vi "Do_channel_mathsPLL.vi"(4 "Output Index":i32, 5 "Channel Values In":string[][](array[string]), 6 "Channel Names":string[](array[string]), 7 "Maths Equation":string) -> (0 "Error String":string, 1 "Channel Values Out":string[][](array[string]), 3 "Results":dbl[](array[numeric]) format="%0.2f")   [LabVIEW 2021]
uses:
  <vilib>/Utility/error.llb/whitespace.ctl
  Globals/ParallelExecutionGlobal.vi
  Data_plotting_vis/Results_plotter_Global.vi
  <vilib>/gmath/NI_Gmath.lvlib
panel:
  out "Numeric":i32
  out "Array":string[](array[string])
  out "Generic Equation":string
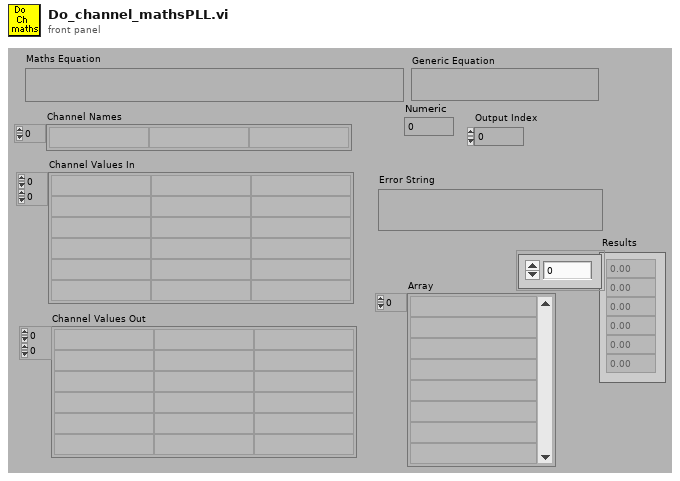
[diagram p1: front panel]
types:
  T1 = cluster{"Tables":i32[][], "Y Values":dbl[], "Variables input decode":i32[], i32[]}[]
  T2 = cluster{"Y Values":dbl[][], "Tables":i32[][][], "Variables input decode":i32[], "Variables output decode":i32[]}
  T3 = cluster{"Tables":i32[][], "Y Values":dbl[], "Variables input decode":i32[], i32[]}
  T4 = typedef "whitespace.ctl" = u16
  T5 = typedef "LVDateTimeRec.ctl" = cluster{"fractional second":dbl, "second":i32, "minute":i32, "hour":i32, "day of month":i32, "month":i32, "year":i32, "day of week":i32, "day of year":i32, "DST":i32}
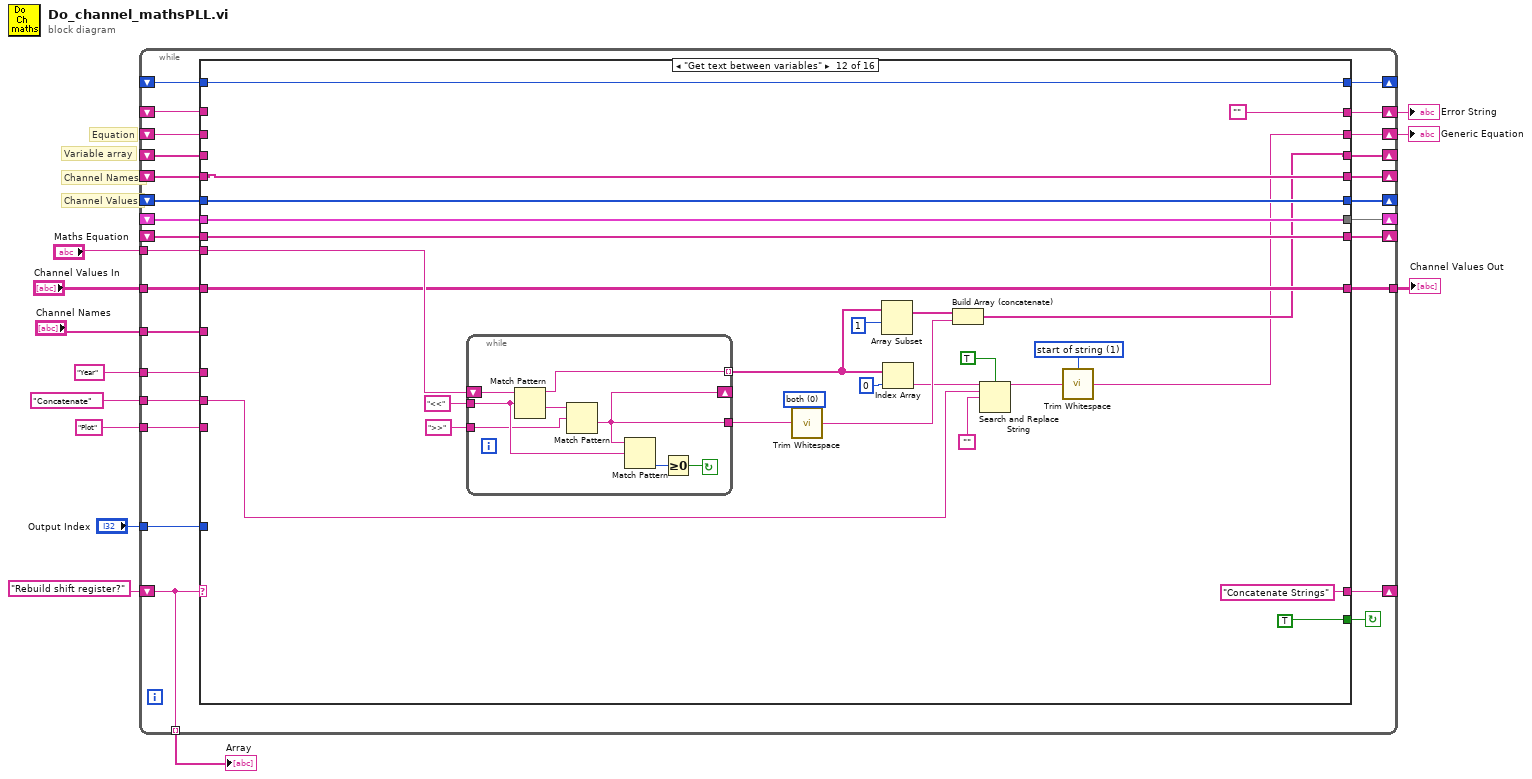
[diagram p0: block diagram]
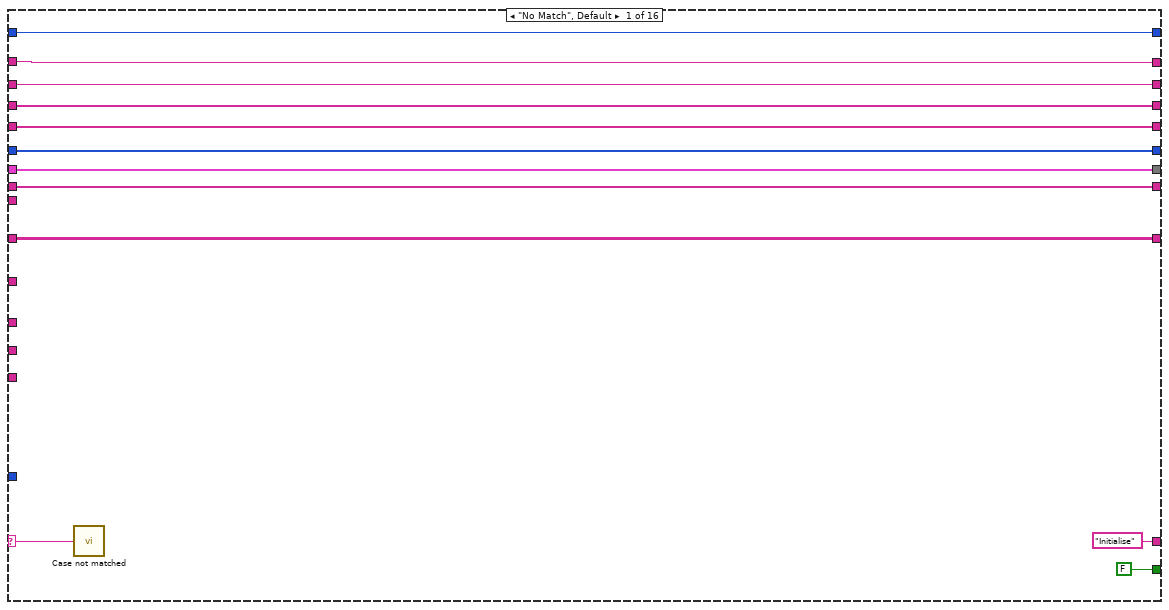
[diagram p2: hidden frame]
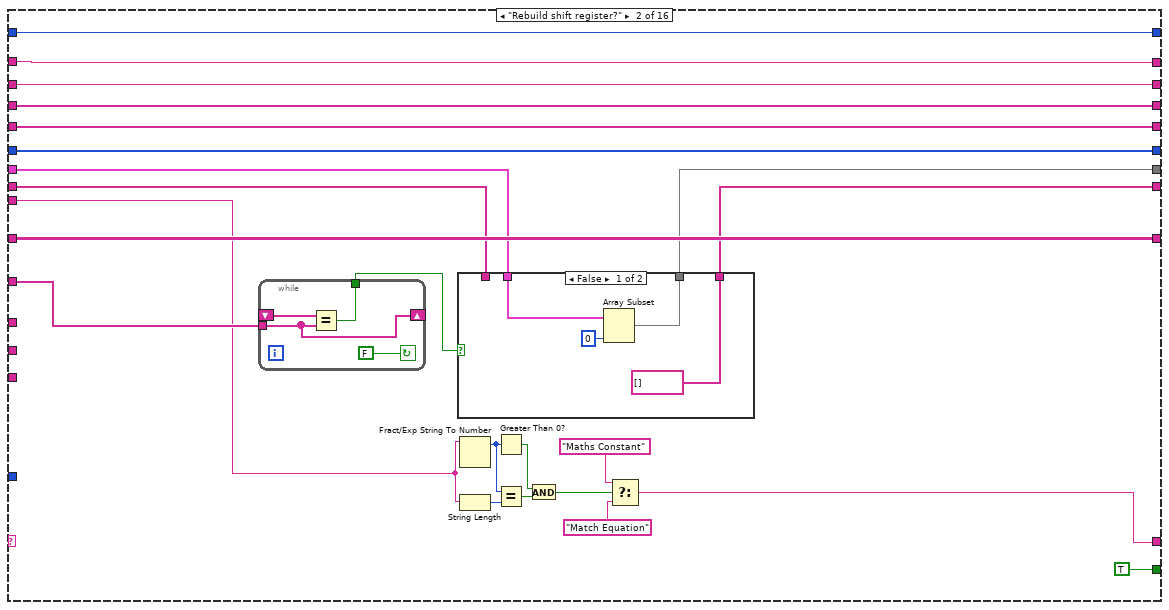
[diagram p3: hidden frame]
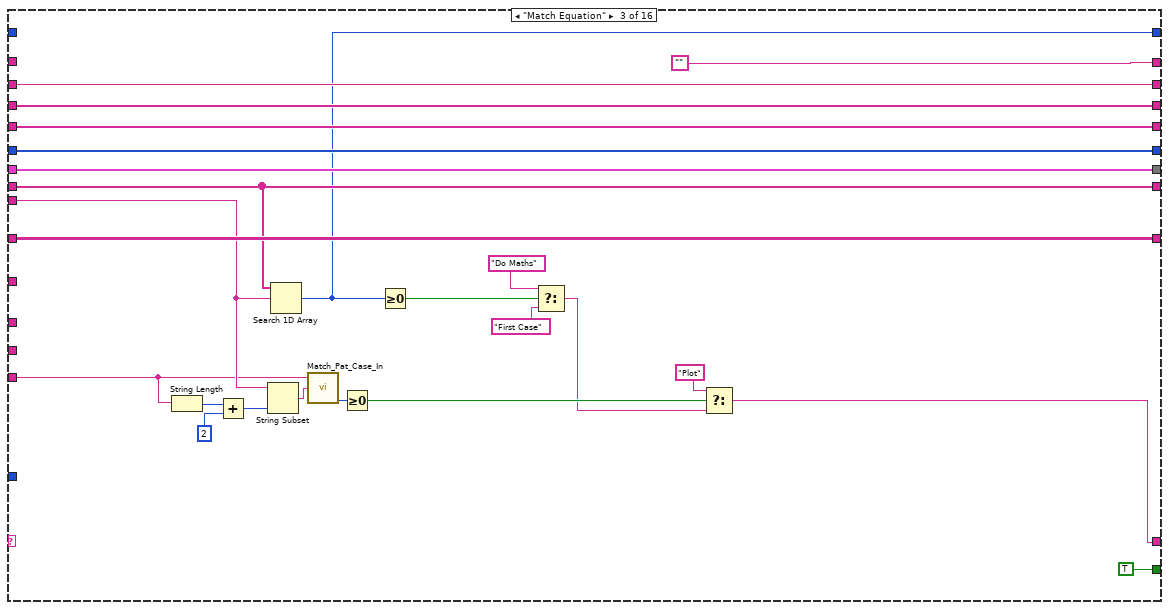
[diagram p5: hidden frame]
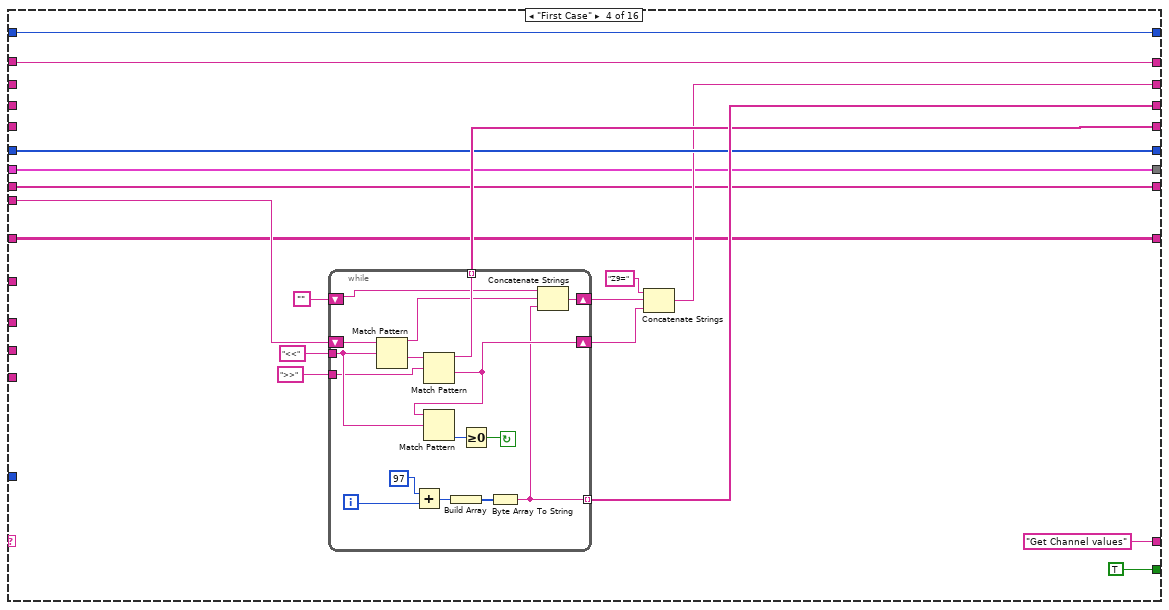
[diagram p6: hidden frame]
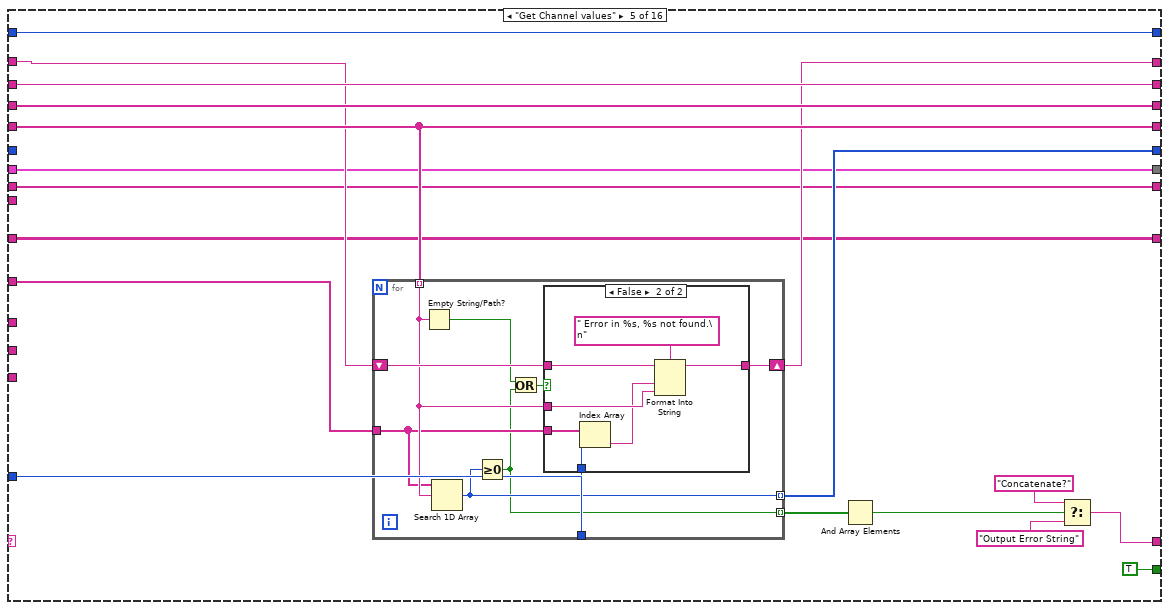
[diagram p7: hidden frame]
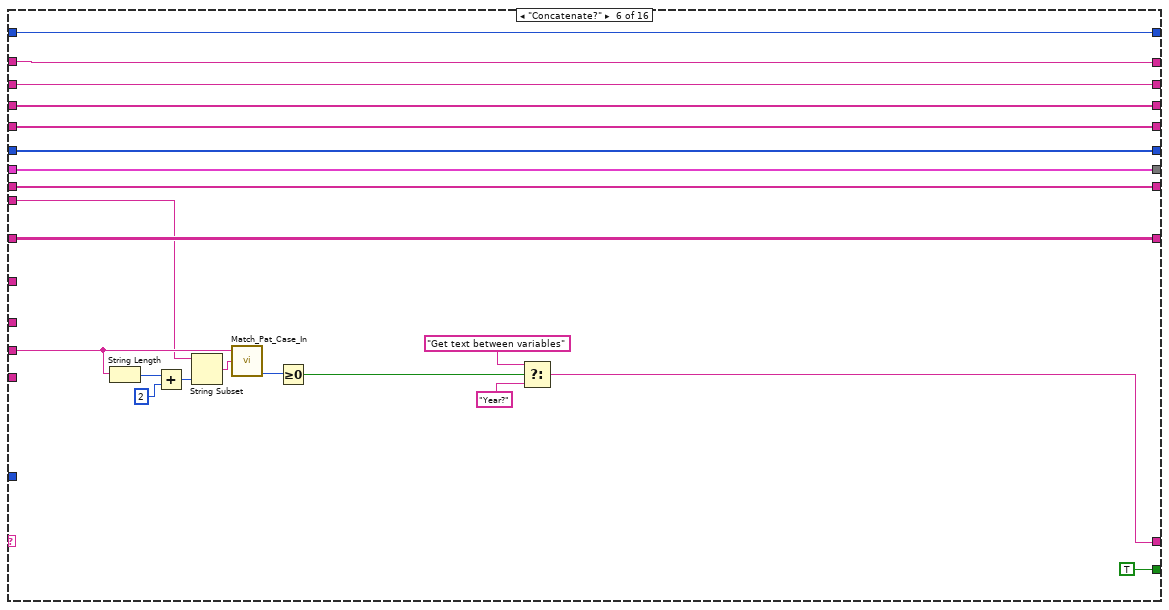
[diagram p9: hidden frame]
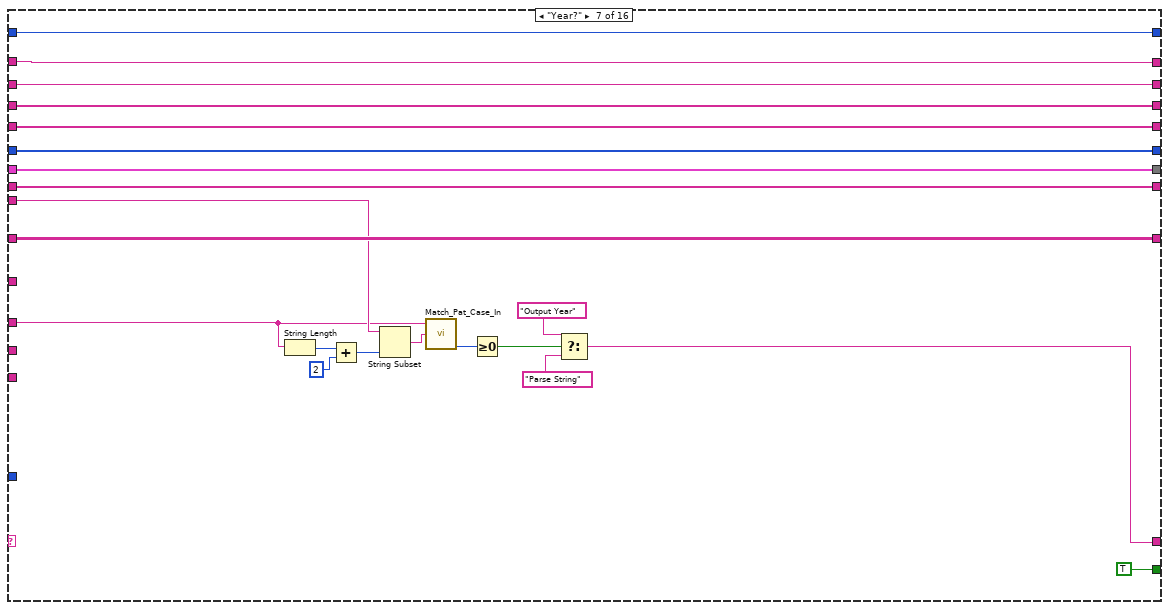
[diagram p10: hidden frame]
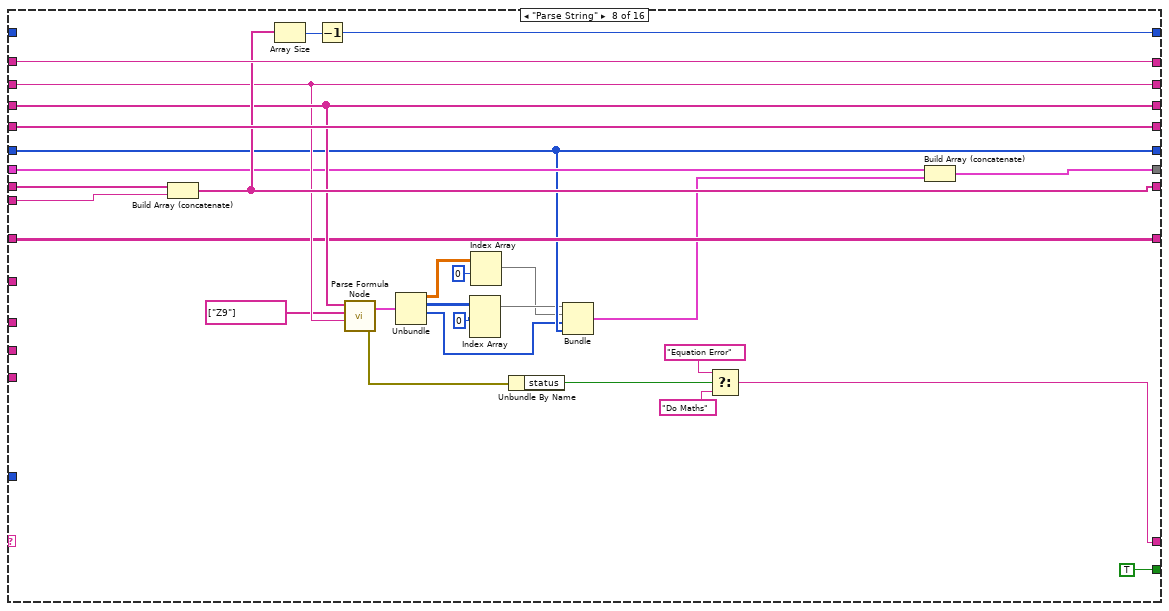
[diagram p11: hidden frame]
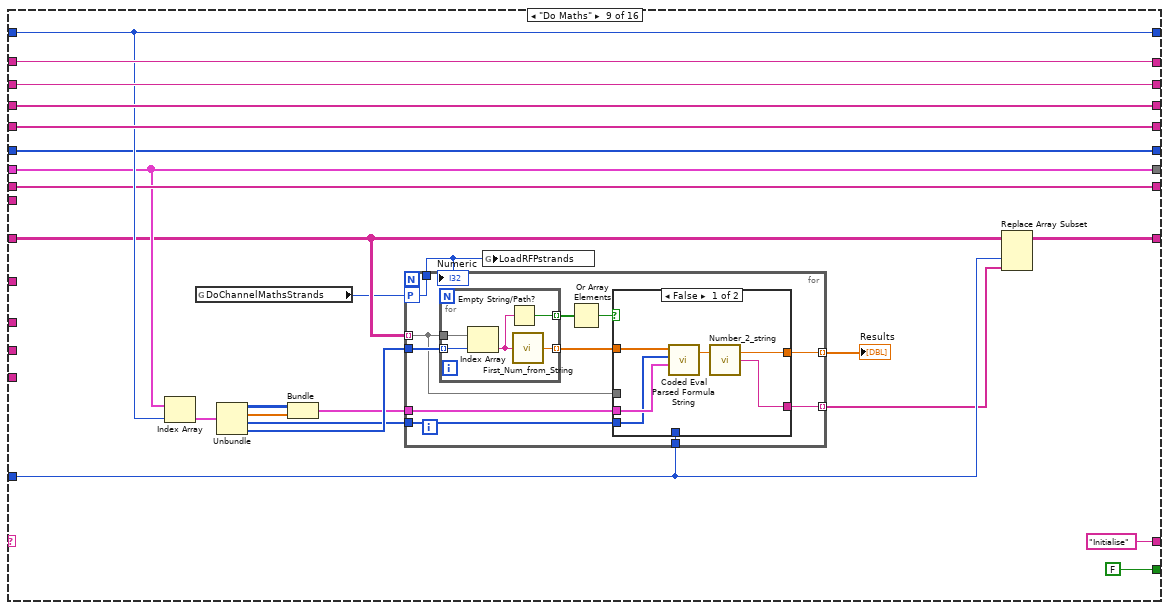
[diagram p12: hidden frame]
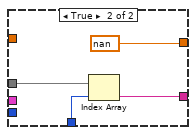
[diagram p13: hidden frame]
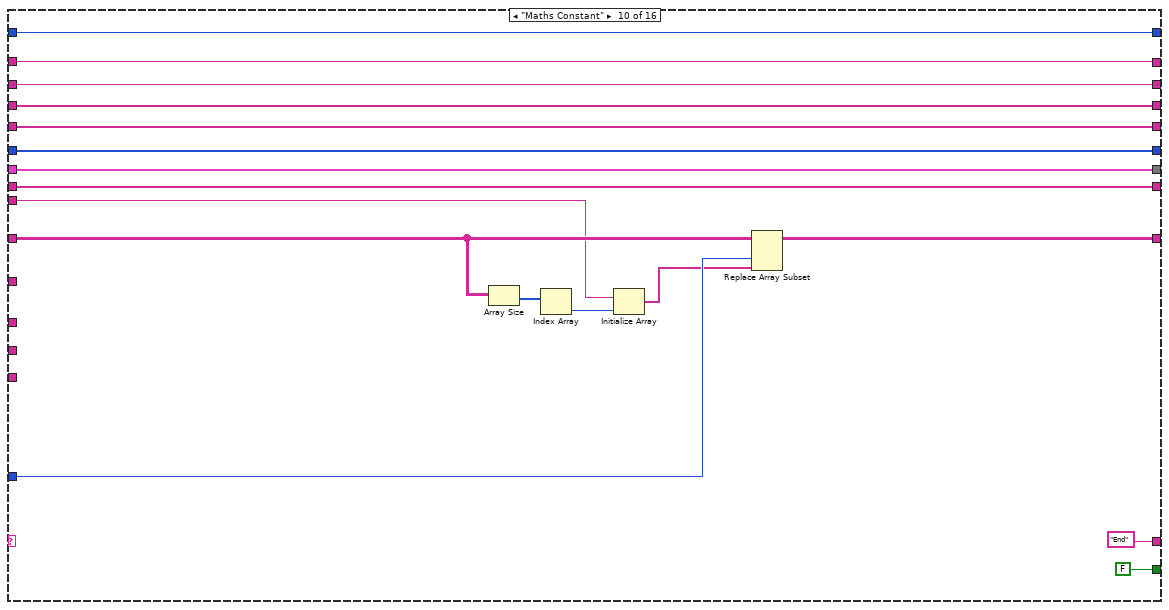
[diagram p14: hidden frame]
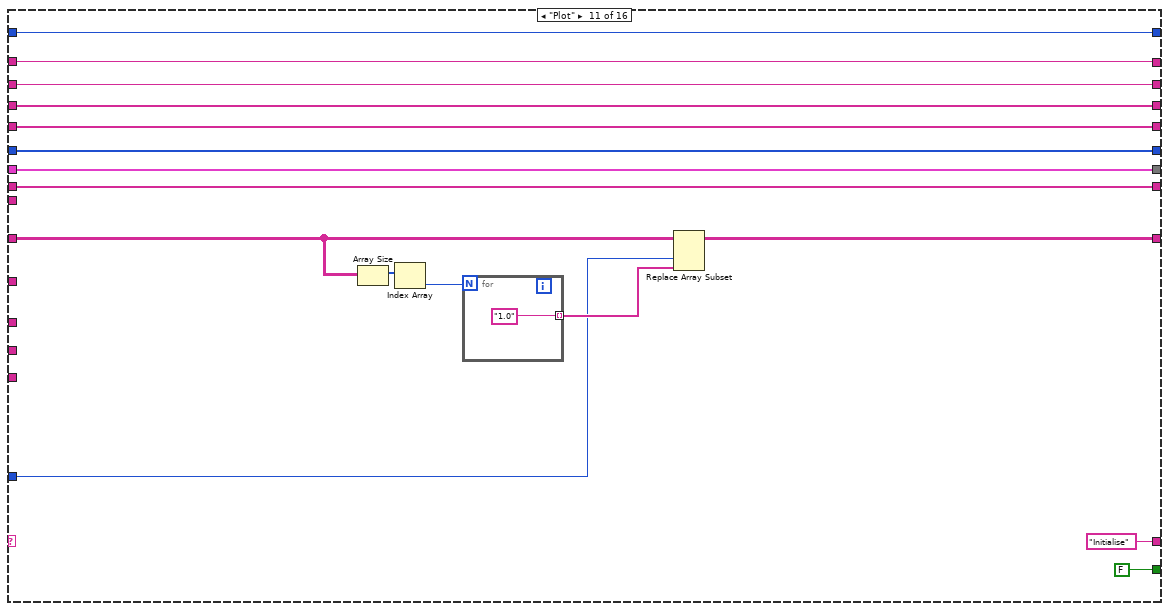
[diagram p15: hidden frame]
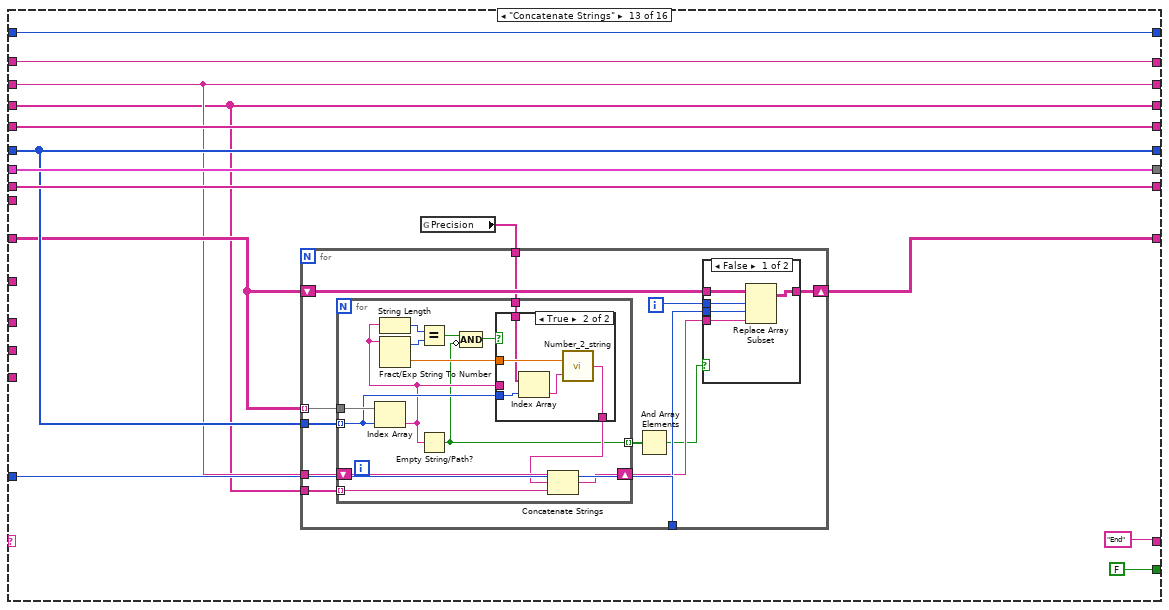
[diagram p16: hidden frame]
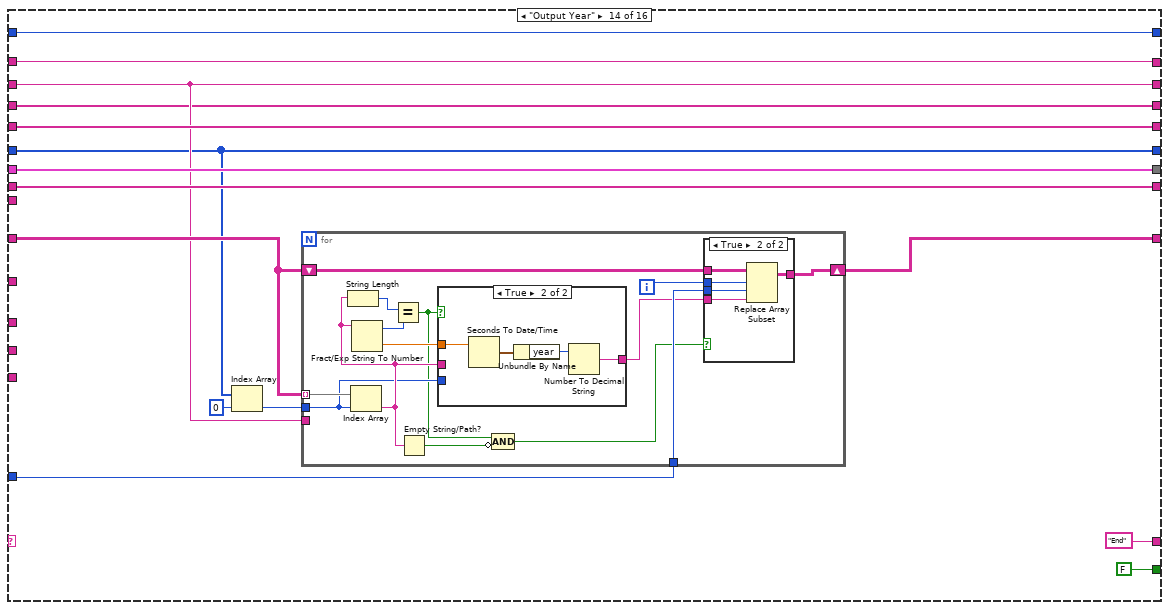
[diagram p19: hidden frame]
diagram:
  # "Channel Names"
  # "Variable array"
  # "Channel Values"
  # "Equation"
  n1 = while {
    tunnel: [w17] -> w6
    tunnel: "Output Index" -> [w18]
    shift-left: _ -> [w19]
    shift-right: [w20] -> _
    shift-left: _ -> [w23]
    shift-right: [w22] -> _
    shift-left: _ -> [w21]
    shift-right: [w24] -> _
    tunnel: "Channel Values In" -> [w25]
    tunnel: "Channel Names" -> [w26]
    tunnel: "Maths Equation" -> [w27]
    shift-left: _ -> [w29]
    shift-right: [w28] -> _
    shift-left: _ -> [w31]
    shift-right: [w30] -> _
    shift-left: _ -> [w33]
    shift-right: [w32] -> _
    shift-left: _ -> [w35]
    shift-right: [w34] -> w8
    shift-left: _ -> [w37]
    shift-right: [w36] -> w9
    shift-left: "Rebuild shift register?" -> [w13]
    shift-right: [w38] -> _
    tunnel: "Concatenate" ("regular expression") -> [w16]
    tunnel: "Plot" ("regular expression") -> [w15]
    tunnel: "Year" ("regular expression") -> [w14]
    tunnel: [w13] -> w1 mode=indexing
    stop <- w39 continue-if-true
    n2 = case shown="\"Get text between variables\"" w13 {
      selector: w13 -> [w40 _ _ _ _ _ _ _ _ _ _ _ _ _ _ _]
      tunnel: [FALSE TRUE TRUE TRUE TRUE TRUE TRUE TRUE FALSE FALSE FALSE TRUE FALSE FALSE TRUE FALSE] -> w39
      tunnel: ["Initialise" w53 w86 "Get Channel values" w145 w178 w208 w234 "Initialise" "End" "Initialise" "Concatenate Strings" "End" "End" "Output Error String" "Initialise"] -> w38
      tunnel: w37 -> [w49 w73 _ w111 w153 w198 w219 w246 w268 w310 w326 _ w376 w429 w459 w472]
      tunnel: [w49 w73 "" w111 w154 w198 w219 w246 w268 w310 w326 "" w376 w429 w458 w472] -> w36
      tunnel: w35 -> [w48 w72 w108 _ w159 w197 w218 w242 w266 w308 w324 _ w368 w422 w461 w482]
      tunnel: [w48 w72 w108 w116 w159 w197 w218 w242 w266 w308 w324 w332 w368 w422 w461 w482] -> w34
      tunnel: w33 -> [w47 w71 w107 _ w158 w196 w217 w243 w267 w309 w325 _ w367 w421 w468 w483]
      tunnel: [w47 w71 w107 w123 w158 w196 w217 w243 w267 w309 w325 w343 w367 w421 w468 w483] -> w32
      tunnel: w31 -> [w46 w70 w106 _ w156 w195 w216 w247 w269 w311 w327 w348 w377 w430 w469 w484]
      tunnel: [w46 w70 w106 w119 w156 w195 w216 w247 w269 w311 w327 w348 w377 w430 w469 w484] -> w30
      tunnel: w29 -> [w45 w69 w105 w118 _ w194 w215 w233 w259 w304 w320 w353 w372 w420 w464 w476]
      tunnel: [w45 w69 w105 w118 w155 w194 w215 w233 w259 w304 w320 w353 w372 w420 w464 w476] -> w28
      tunnel: w27 -> [_ w52 w92 w124 _ w182 w202 w220 _ w298 _ w355 _ _ w460 _]
      tunnel: w26 -> [_ w66 _ _ w157 _ _ _ _ _ _ _ _ _ _ w474]
      tunnel: w25 -> [w41 w67 w103 w112 w149 w189 w207 w238 w251 w301 w316 w349 w371 w425 w463 w475]
      tunnel: [w44 w64 w104 w115 w152 w193 w214 w239 w263 w305 w321 w352 w373 w426 w465 w479] -> w24
      tunnel: w23 -> [w43 w62 w102 w114 w151 w192 w213 w245 w264 w306 w322 w351 w374 w427 w466 w480]
      tunnel: [w43 w61 w102 w114 w151 w192 w213 w244 w264 w306 w322 w351 w374 w427 w466 w480] -> w22
      tunnel: w21 -> [w44 w63 w104 w115 w152 w193 w214 w241 w263 w305 w321 w352 w373 w426 w465 w479]
      tunnel: [w42 w68 w101 w113 w150 w191 w212 w240 w265 w307 w323 w350 w375 w428 w467 w481] -> w20
      tunnel: w19 -> [w42 w68 _ w113 w150 w191 w212 _ w265 w307 w323 w350 w375 w428 w467 w481]
      tunnel: w18 -> [_ _ _ _ w143 _ _ _ w257 w302 w317 _ w370 w424 _ w478]
      tunnel: [w41 w67 w103 w112 w149 w189 w207 w238 w258 w303 w319 w349 w369 w423 w463 w477] -> w17
      tunnel: w16 -> [_ _ _ _ _ w188 _ _ _ _ _ w337 _ _ _ _]
      tunnel: w15 -> [_ _ w91 _ _ _ _ _ _ _ _ _ _ _ _ _]
      tunnel: w14 -> [_ _ _ _ _ _ w199 _ _ _ _ _ _ _ _ _]
      frame "No Match", Default {
        n3 = call "Case not matched.vi"("Case Name not Matched"=w40) -> ()
      }
      frame "Rebuild shift register?" {
        n4 = while {
          shift-right: [w83] -> _
          shift-left: _ -> [w84]
          tunnel: w66 -> [w83]
          tunnel: [w82] -> w65
          stop <- FALSE continue-if-true
          n5 = Equal?(x=w84, y=w83) -> (x = y?=w82:bool)
        }
        n6 = case shown="False" w65 {
          tunnel: [w76 w80] -> w64
          tunnel: w63 -> [w78 w80]
          tunnel: w62 -> [_ w79]
          tunnel: [string[] [] w79] -> w61
          frame False {
            n7 = Array Subset(array=w78, length=0) -> (w76:T1)  [unwired: 1 in]
          }
          frame True {
          }
        }
        n8 = Fract/Exp String To Number(string=w52) -> (offset past number=w60:i32)  [unwired: 3 in, 1 out]
        n9 = String Length(string=w52) -> (length=w59:i32)
        n10 = Greater Than 0?(x=w60) -> (x > 0?=w57:bool)
        n11 = Equal?(x=w60, y=w59) -> (x = y?=w58:bool)
        n12 = And(x=w57, y=w58) -> (x .and. y?=w56:bool)
        n13 = Select(t="Maths Constant", s=w56, f="Match Equation") -> (s? t:f=w53:string)
      }
      frame "Match Equation" {
        n14 = String Length(string=w91) -> (length=w93:i32)
        n15 = Add(x=w93, y=2) -> (x+y=w95:i32)
        n16 = String Subset(string=w92, length (rest)=w95) -> (substring=w96:string)  [unwired: 1 in]
        n17 = Search 1D Array(1D array=w102, element=w92) -> (index of element=w101:i32)  [unwired: 1 out]
        n18 = call "Match_Pat_Case_In.vi"("String to match"=w91, "String"=w96) -> ("offset past match"=w89:i32)  [unwired: 1 in, 3 out]
        n19 = Greater Or Equal To 0?(x=w89) -> (x >= 0?=w88:bool)
        n20 = Greater Or Equal To 0?(x=w101) -> (x >= 0?=w100:bool)
        n21 = Select(t="Do Maths", s=w100, f="First Case") -> (s? t:f=w87:string)
        n22 = Select(t="Plot", s=w88, f=w87) -> (s? t:f=w86:string)
      }
      frame "First Case" {
        n23 = while {
          shift-left: "" -> [w129]
          shift-right: [w130] -> w121
          tunnel: [w131] -> w123 mode=indexing
          tunnel: [w137] -> w119 mode=indexing
          shift-left: w124 -> [w142]
          shift-right: [w140] -> w120
          tunnel: "<<" ("regular expression") -> [w128]
          tunnel: ">>" ("regular expression") -> [w127]
          i -> [w133]
          stop <- w138 continue-if-true
          n24 = Match Pattern(string=w142, regular expression=w128) -> (before substring=w132:string, after substring=w141:string)  [unwired: 3 out]
          n25 = Add(x=97, y=w133) -> (x+y=w135:i32)
          n26 = Match Pattern(string=w141, regular expression=w127) -> (before substring=w137:string, after substring=w140:string)  [unwired: 3 out]
          n27 = Match Pattern(string=w140, regular expression=w128) -> (offset past match=w139:i32)  [unwired: 4 out]
          n28 = Build Array(w135) -> (w136:i32[])
          n29 = Greater Or Equal To 0?(x=w139) -> (x >= 0?=w138:bool)
          n30 = Byte Array To String(unsigned byte array=w136) -> (string=w131:string)
          n31 = Concatenate Strings(w129, w132, w131) -> (w130:string)
        }
        n32 = Concatenate Strings("Z9=" ("Substring"), w121, w120) -> (w116:string)
      }
      frame "Get Channel values" {
        n33 = for {
          tunnel: w157 -> [w164]
          tunnel: w156 -> [w166] mode=indexing
          tunnel: [w167] -> w155 mode=indexing
          shift-right: [w168] -> w154
          shift-left: w153 -> [w169]
          tunnel: [w161] -> w148 mode=indexing
          tunnel: w143 -> [w163]
          n34 = Empty String/Path?(string/path=w166) -> (empty?=w162:bool)
          n35 = Search 1D Array(1D array=w164, element=w166) -> (index of element=w167:i32)  [unwired: 1 out]
          n36 = Greater Or Equal To 0?(x=w167) -> (x >= 0?=w161:bool)
          n37 = Or(x=w162, y=w161) -> (x .or. y?=w165:bool)
          n38 = case shown="False" w165 {
            tunnel: w166 -> [_ w177]
            tunnel: w169 -> [w170 w175]
            tunnel: [w170 w174] -> w168
            tunnel: w164 -> [_ w173]
            tunnel: w163 -> [_ w172]
            frame True {
            }
            frame False {
              n39 = Index Array(array=w173, index=w172) -> (element=w171:string)
              n40 = Format Into String(format string=" Error in %s, %s not found.\n" ("Format String"), initial string=w175, w171, w177) -> (resulting string=w174:string)  [unwired: 1 in, 1 out]
            }
          }
        }
        n41 = And Array Elements(Boolean array=w148) -> (logical AND=w147:bool)
        n42 = Select(t="Concatenate?", s=w147, f="Output Error String") -> (s? t:f=w145:string)
      }
      frame "Concatenate?" {
        n43 = String Length(string=w188) -> (length=w187:i32)
        n44 = Add(x=w187, y=2) -> (x+y=w185:i32)
        n45 = String Subset(string=w182, length (rest)=w185) -> (substring=w184:string)  [unwired: 1 in]
        n46 = call "Match_Pat_Case_In.vi"("String to match"=w188, "String"=w184) -> ("offset past match"=w190:i32)  [unwired: 1 in, 3 out]
        n47 = Greater Or Equal To 0?(x=w190) -> (x >= 0?=w180:bool)
        n48 = Select(t="Get text between variables" ("regular expression"), s=w180, f="Year?" ("regular expression")) -> (s? t:f=w178:string)
      }
      frame "Year?" {
        n49 = String Length(string=w199) -> (length=w206:i32)
        n50 = Add(x=w206, y=2) -> (x+y=w204:i32)
        n51 = String Subset(string=w202, length (rest)=w204) -> (substring=w203:string)  [unwired: 1 in]
        n52 = call "Match_Pat_Case_In.vi"("String to match"=w199, "String"=w203) -> ("offset past match"=w211:i32)  [unwired: 1 in, 3 out]
        n53 = Greater Or Equal To 0?(x=w211) -> (x >= 0?=w201:bool)
        n54 = Select(t="Output Year" ("regular expression"), s=w201, f="Parse String" ("regular expression")) -> (s? t:f=w208:string)
      }
      frame "Parse String" {
        n55 = Build Array (concatenate)(w245, w220) -> (w244:string[])
        n56 = Array Size(array=w244) -> (size(s)=w231:i32)
        n57 = Decrement(x=w231) -> (x-1=w240:i32)
        n58 = call <vilib>:"Parse Formula Node.vi"("formula"=w242, "Variables Output"=string[] ["Z9"], "Variables Input"=w243) -> ("error out"=w221:errorcluster, "Parsed Formula Node"=w230:T2)  [unwired: 1 in]
        n59 = Unbundle(w230) -> ("Y Values"=w229:dbl[][], "Tables"=w226:i32[][][], "Variables input decode"=w223:i32[])  [unwired: 1 out]
        n60 = Index Array(array=w226, index (dim 0)=0 ("Index")) -> (element=w225:i32[][])  [unwired: 2 in]
        n61 = Index Array(array=w229, index (row)=0 ("Index")) -> (element=w224:dbl[])  [unwired: 1 in]
        n62 = Unbundle By Name(w221) -> ("status"=w237:bool)
        n63 = Bundle("Tables"=w225, "Y Values"=w224, "Variables input decode"=w223, w233) -> (w222:T3)  [unwired: 1 out]
        n64 = Select(t="Equation Error", s=w237, f="Do Maths") -> (s? t:f=w234:string)
        n65 = Build Array (concatenate)(w241, w222) -> (w239:T1)
      }
      frame "Do Maths" {
        n66 = Index Array(array=w263, index=w265) -> (element=w262:T3)
        n67 = global read "ParallelExecutionGlobal.vi" "DoChannelMathsStrands"() -> (w250:i32)
        n68 = Unbundle(w262) -> ("Tables"=w261:i32[][], "Y Values"=w260:dbl[], "Variables input decode"=w255:i32[], w256:i32[])
        n69 = Bundle("Tables"=w261, "Y Values"=w260) -> (w254:cluster{"Tables":i32[][], "Y Values":dbl[]})  [unwired: 1 out]
        n70 = for {
          tunnel: w251 -> [w275] mode=indexing
          tunnel: w256 -> [w282]
          tunnel: w254 -> [w280]
          tunnel: w255 -> [w279]
          tunnel: [w276] -> w253 mode=indexing
          tunnel: w257 -> [w274]
          tunnel: [w273] -> w252 mode=indexing
          workers-P: w250 -> [w272]
          tunnel: [w272] -> w249
          n71 = for {
            tunnel: w275 -> [w296]
            tunnel: w282 -> [w295] mode=indexing
            tunnel: [w292] -> w281 mode=indexing
            tunnel: [w294] -> w278 mode=indexing
            n72 = Index Array(array=w296, index=w295) -> (element=w293:string)
            n73 = Empty String/Path?(string/path=w293) -> (empty?=w294:bool)
            n74 = call "First_Num_from_String.vi"("string"=w293) -> ("number"=w292:dbl)
          }
          n75 = Or Array Elements(Boolean array=w278) -> (logical OR=w277:bool)
          n76 = case shown="False" w277 {
            tunnel: w281 -> [w287 _]
            tunnel: w280 -> [w286 _]
            tunnel: w279 -> [w285 _]
            tunnel: [w284 w289] -> w276
            tunnel: w275 -> [_ w291]
            tunnel: w274 -> [_ w290]
            tunnel: [w283 nan ("y value")] -> w273
            frame False {
              n77 = call <vilib>:"Coded Eval Parsed Formula String.vi"("Parsed Formula"=w286, "Variables"=w285, "X Values"=w287) -> ("y value"=w283:dbl)  [unwired: 1 in, 1 out]
              n78 = call "Number_2_string.vi"("number"=w283) -> ("String"=w284:string)  [unwired: 1 in]
            }
            frame True {
              n79 = Index Array(array=w291, index=w290) -> (element=w289:string)
            }
          }
        }
        "Results" <- w252
        "Numeric" <- w249
        n80 = global write "ParallelExecutionGlobal.vi" "LoadRFPstrands"(w249) -> ()
        n81 = Replace Array Subset(array=w251, new element=w253, index (col)=w257) -> (w258:string[][])  [unwired: 1 in]
      }
      frame "Maths Constant" {
        n82 = Array Size(array=w301) -> (size(s)=w300:i32[])
        n83 = Index Array(array=w300) -> (element=w299:i32)  [unwired: 1 in]
        n84 = Initialize Array(w298, w299) -> (w297:string[])
        n85 = Replace Array Subset(array=w301, new element=w297, index (col)=w302) -> (w303:string[][])  [unwired: 1 in]
      }
      frame "Plot" {
        n86 = Array Size(array=w316) -> (size(s)=w315:i32[])
        n87 = Index Array(array=w315) -> (element=w314:i32)  [unwired: 1 in]
        n88 = for {
          N: w314 -> [_]
          tunnel: ["1.0"] -> w318 mode=indexing
        }
        n89 = Replace Array Subset(array=w316, new element=w318, index (col)=w317) -> (w319:string[][])  [unwired: 1 in]
      }
      frame "Get text between variables" {
        w331 = T4 1 items=["both", "start of string", "end of string"] ("location (both)")
        w333 = T4 0 items=["both", "start of string", "end of string"] ("location (both)")
        n90 = while {
          shift-left: w355 -> [w365]
          shift-right: [w360] -> _
          tunnel: [w361] -> w346 mode=indexing
          tunnel: [w360] -> w342
          tunnel: "<<" ("regular expression") -> [w359]
          tunnel: ">>" ("regular expression") -> [w358]
          stop <- w362 continue-if-true
          n91 = Match Pattern(string=w365, regular expression=w359) -> (before substring=w361:string, after substring=w364:string)  [unwired: 3 out]
          n92 = Match Pattern(string=w364, regular expression=w358) -> (after substring=w360:string)  [unwired: 4 out]
          n93 = Match Pattern(string=w360, regular expression=w359) -> (offset past match=w363:i32)  [unwired: 4 out]
          n94 = Greater Or Equal To 0?(x=w363) -> (x >= 0?=w362:bool)
        }
        n95 = call <vilib>:"Trim Whitespace.vi"("string"=w342, "location (both)"=w333) -> ("trimmed string"=w341:string)
        n96 = Array Subset(array=w346, index=1) -> (w345:string[])  [unwired: 1 in]
        n97 = Index Array(array=w346, index=0) -> (element=w338:string)
        n98 = Build Array (concatenate)(w345, w341) -> (w343:string[])
        n99 = Search and Replace String(case sensitive?=TRUE ("ignore case? (F)"), input string=w338, search string=w337, replace string="") -> (result string=w334:string)  [unwired: 4 in, 3 out]
        n100 = call <vilib>:"Trim Whitespace.vi"("string"=w334, "location (both)"=w331) -> ("trimmed string"=w332:string)
      }
      frame "Concatenate Strings" {
        n101 = global read "Results_plotter_Global.vi" "Precision"() -> (w366:string[])
        n102 = for {
          tunnel: w371 -> [w391] mode=indexing
          shift-right: [w388] -> w369
          shift-left: w371 -> [w389]
          tunnel: w372 -> [w390]
          tunnel: w370 -> [w386]
          tunnel: w368 -> [w385]
          tunnel: w367 -> [w384]
          tunnel: w366 -> [w383]
          i -> [w387]
          n103 = for {
            tunnel: w391 -> [w411]
            tunnel: w390 -> [w404] mode=indexing
            shift-right: [w402] -> w382
            shift-left: w385 -> [w410]
            tunnel: w384 -> [w409] mode=indexing
            tunnel: w383 -> [w403]
            tunnel: [w399] -> w381 mode=indexing
            n104 = Index Array(array=w411, index=w404) -> (element=w401:string)
            n105 = String Length(string=w401) -> (length=w408:i32)
            n106 = Fract/Exp String To Number(string=w401) -> (offset past number=w407:i32, number=w406:dbl)  [unwired: 3 out]
            n107 = Equal?(x=w408, y=w407) -> (x = y?=w400:bool)
            n108 = Empty String/Path?(string/path=w401) -> (empty?=w399:bool)
            n109 = Compound Arithmetic op=AND(w400, invert w399) -> (w398:bool)
            n110 = case shown="True" w398 {
              tunnel: w406 -> [_ w417]
              tunnel: [w412 w416] -> w405
              tunnel: w401 -> [w412 _]
              tunnel: w404 -> [_ w415]
              tunnel: w403 -> [_ w414]
              frame False {
              }
              frame True {
                n111 = Index Array(array=w414, index=w415) -> (element=w413:string)
                n112 = call "Number_2_string.vi"("precision"=w413, "number"=w417) -> ("String"=w416:string)
              }
            }
            n113 = Concatenate Strings(w410, w405, w409) -> (w402:string)
          }
          n114 = And Array Elements(Boolean array=w381) -> (logical AND=w380:bool)
          n115 = case shown="False" w380 {
            tunnel: w389 -> [w396 w397]
            tunnel: [w395 w397] -> w388
            tunnel: w387 -> [w394 _]
            tunnel: w386 -> [w393 _]
            tunnel: w382 -> [w392 _]
            frame False {
              n116 = Replace Array Subset(array=w396, new element=w392, index (row)=w394, index (col)=w393) -> (w395:string[][])
            }
            frame True {
            }
          }
        }
      }
      frame "Output Year" {
        n117 = Index Array(array=w420, index=0) -> (element=w418:i32)
        n118 = for {
          tunnel: w425 -> [w446] mode=indexing
          shift-right: [w444] -> w423
          shift-left: w425 -> [w445]
          tunnel: w424 -> [w442]
          tunnel: w422 -> [_]
          tunnel: w418 -> [w437]
          i -> [w443]
          n119 = Index Array(array=w446, index=w437) -> (element=w438:string)
          n120 = String Length(string=w438) -> (length=w441:i32)
          n121 = Fract/Exp String To Number(string=w438) -> (offset past number=w440:i32, number=w439:dbl)  [unwired: 3 out]
          n122 = Equal?(x=w441, y=w440) -> (x = y?=w434:bool)
          n123 = Empty String/Path?(string/path=w438) -> (empty?=w435:bool)
          n124 = case shown="True" w434 {
            tunnel: w439 -> [_ w451]
            tunnel: [w447 w448] -> w436
            tunnel: w438 -> [w447 _]
            tunnel: w437 -> [_ _]
            frame False {
            }
            frame True {
              n125 = Seconds To Date/Time(time stamp (now)=w451) -> (date time rec=w450:T5)  [unwired: 1 in]
              n126 = Unbundle By Name(w450) -> ("year"=w449:i32)
              n127 = Number To Decimal String(number=w449) -> (decimal integer string=w448:string)  [unwired: 1 in]
            }
          }
          n128 = Compound Arithmetic op=AND(w434, invert w435) -> (w433:bool)
          n129 = case shown="True" w433 {
            tunnel: w445 -> [w452 w457]
            tunnel: [w452 w456] -> w444
            tunnel: w443 -> [_ w455]
            tunnel: w442 -> [_ w454]
            tunnel: w436 -> [_ w453]
            frame False {
            }
            frame True {
              n130 = Replace Array Subset(array=w457, new element=w453, index (row)=w455, index (col)=w454) -> (w456:string[][])
            }
          }
        }
      }
      frame "Equation Error" {
        n131 = Format Into String(format string="There is an error in the Maths Equation %s. The full equation is %s", initial string=w459, w461, w460) -> (resulting string=w458:string)  [unwired: 1 in, 1 out]
      }
      frame "Output Error String" {
        n132 = Array Size(array=w474) -> (size(s)=w473:i32)
        n133 = for {
          N: w473 -> [_]
          shift-right: [w490] -> w477
          shift-left: w475 -> [w491]
          tunnel: w478 -> [w488]
          tunnel: w472 -> [w487]
          i -> [w489]
          n134 = Replace Array Subset(array=w491, new element=w487, index (row)=w489, index (col)=w488) -> (w490:string[][])
        }
      }
    }
  }
  "Error String" <- w9
  "Generic Equation" <- w8
  "Channel Values Out" <- w6
  "Array" <- w1
